vi "WriteHeader+MzArray(AnalyzeV75).vi"(8 "error in (no error)":errorcluster, 11 "ImageConvParams":T1={"File Header"={"Start Position"=[], "StepWidth"=[0.05, 0.05], "Dimension"=[], "SpecLength"=10000}, "mzCali."=[0.0, 1.0, 0.0], "m/z_Array"=[0.0, 1.0, 0.0], "SampleRate"=0.0, "TrigDelay"=0.0, "file refnum"=refnum, "file path"=path "", "PeakOI"=[], "Binning"={"Enable"=FALSE, "BinType"=enum."ByScreen", "BinWidth"=0.5, "Maximum"=0.0, "Minimum"=0.0}} {"SampleRate" items=["50MS/s"=50000000.0, "100MS/s"=100000000.0, "125MS/s"=125000000.0, "200MS/s"=200000000.0, "250MS/s"=250000000.0, "500MS/s"=500000000.0, "1GS/s"=1000000000.0, "1.6GS/s"=1600000000.0, "2GS/s"=2000000000.0, "4GS/s"=4000000000.0]}) -> (0 "error out":errorcluster)   [LabVIEW 2014]
uses:
  ProcessMethods/BioMapConversion/BioMAPWriterCoreParams.ctl
  Files/BinaryHeader.ctl
  ControlDef/SampleRateSelector.ctl
  ProcessMethods/Binning/BinType.ctl
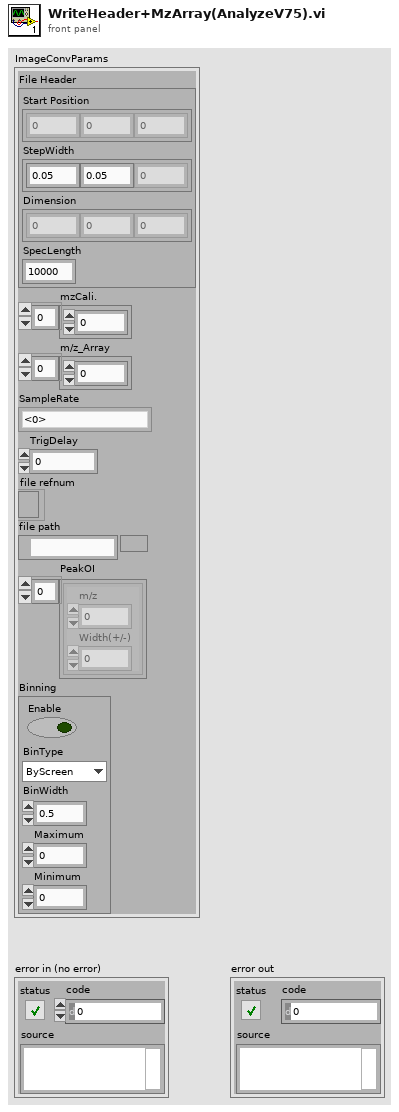
[diagram p1: front panel]
types:
  T1 = typedef "BioMAPWriterCoreParams.ctl" = cluster{"File Header":T2, "mzCali.":dbl[], "m/z_Array":dbl[], "SampleRate":T3, "TrigDelay":dbl, "file refnum":refnum<file>, "file path":path, "PeakOI":cluster{"m/z":dbl, "Width(+/-)":dbl}[], "Binning":cluster{"Enable":bool, "BinType":T4, "BinWidth":dbl, "Maximum":dbl, "Minimum":dbl}}
  T2 = typedef "BinaryHeader.ctl" = cluster{"Start Position":dbl[], "StepWidth":dbl[], "Dimension":i32[], "SpecLength":i32}
  T3 = typedef "SampleRateSelector.ctl" = dbl
  T4 = typedef "BinType.ctl" = enum16{"ByTime", "ByScreen", "ByMass", "ToUnitMass"}
  T5 = cluster{"Dimension":u16, "SpecDepth":u16, "x dimension":u16, "y dimension":u16, "z dimension":u16}
  T6 = cluster{"Dimension 1":sgl, "Dimension 2":sgl, "Dimension 3":sgl, "Dimension 4":sgl, "Dimension 5":sgl, "Dimension 6":sgl, "Dimension 7":sgl, "Dimension 8":sgl}
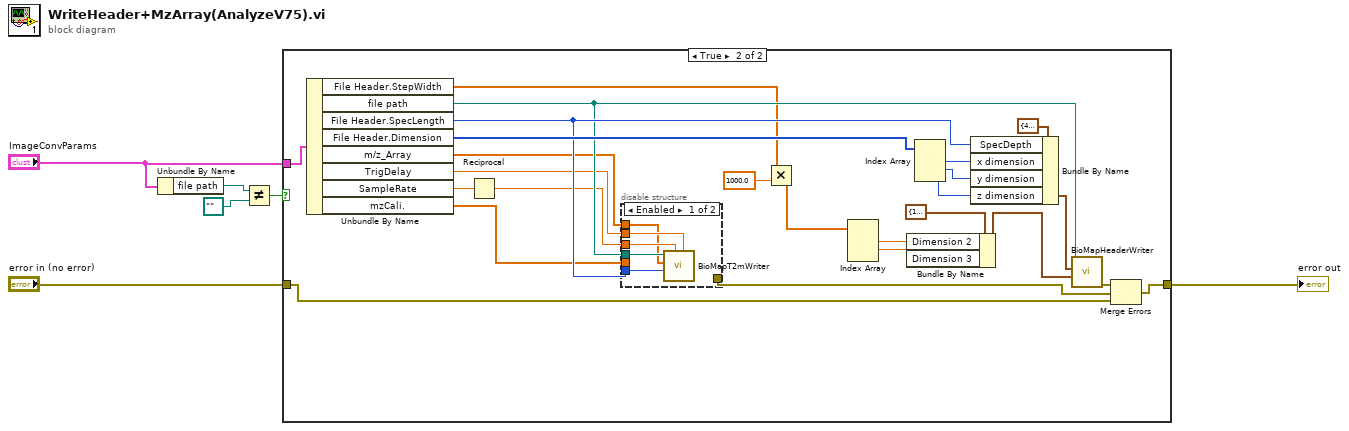
[diagram p0: block diagram]
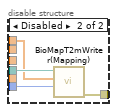
[diagram p3: hidden frame]
diagram:
  n1 = Unbundle By Name("ImageConvParams") -> ("file path"=w6:path)
  n2 = Not Equal?(x=w6, y=path "" ("file path")) -> (x != y?=w4:bool)
  n3 = case shown="True" w4 {
    tunnel: "error in (no error)" -> [w7 w26]
    tunnel: "ImageConvParams" -> [_ w20]
    tunnel: [w7 w19] -> w2
    frame False {
    }
    frame True {
      n4 = Unbundle By Name(w20) -> ("File Header.StepWidth"=w13:dbl[], "file path"=w23:path, "File Header.SpecLength"=w24:i32, "File Header.Dimension"=w25:i32[], "m/z_Array"=w17:dbl[], "TrigDelay"=w16:dbl, "SampleRate"=w22:T3, "mzCali."=w15:dbl[])
      n5 = Reciprocal(x=w22) -> (1/x=w21:T3)
      n6 = disable-structure shown="Enabled" {
        disable-tunnel: w15 -> [_ _]
        disable-tunnel: w24 -> [w37 w38]
        disable-tunnel: w23 -> [w36 w40]
        disable-tunnel: w21 -> [w35 _]
        disable-tunnel: w16 -> [w34 _]
        disable-tunnel: [_ w41] -> w18
        disable-tunnel: w17 -> [w33 w39]
        frame Enabled {
          n7 = call "BioMapT2mWriter.vi"("TrigDelay"=w34, "time bin (s)"=w35, "SpecDepth"=w37, "mzArray"=w33, "image file path"=w36) -> ()  [unwired: 6 in, 1 out]
        }
        frame Disabled {
          n8 = call "BioMapT2mWriter(Mapping).vi"("SpecLength"=w38, "mzArray"=w39, "image file path"=w40) -> ("error out"=w41:errorcluster)  [unwired: 8 in]
        }
      }
      n9 = Multiply(x=w13, y=1000.0) -> (x*y=w9:dbl[])
      n10 = Index Array(array=w9) -> (element #1=w12:dbl, element #2=w11:dbl)  [unwired: 3 in, 1 out]
      n11 = Bundle By Name(cluster=T6 {"Dimension 1"=1.0, "Dimension 2"=1.0, "Dimension 3"=1.0, "Dimension 4"=1.0, "Dimension 5"=0.0, "Dimension 6"=0.0, "Dimension 7"=0.0, "Dimension 8"=0.0} ("Pixel Dimension"), "Dimension 2"=w12, "Dimension 3"=w11) -> (w14:T6)
      n12 = Index Array(array=w25) -> (element #1=w28:i32, element #2=w27:i32, element #3=w10:i32)  [unwired: 3 in]
      n13 = Bundle By Name(cluster=T5 {"Dimension"=4, "SpecDepth"=0, "x dimension"=0, "y dimension"=0, "z dimension"=1} ("Dimensions"), "SpecDepth"=w24, "x dimension"=w28, "y dimension"=w27, "z dimension"=w10) -> (w32:T5)
      n14 = call "BioMapHeaderWriter.vi"("Pixel Dimension"=w14, "Dimensions"=w32, "image file path"=w23) -> ("error out"=w29:errorcluster)  [unwired: 8 in]
      n15 = Merge Errors(w29, w18, w26) -> (w19:errorcluster)
    }
  }
  "error out" <- w2
